vi "Galobal variable_TI.vi"() -> ()   [LabVIEW 2015]
panel:
  in  "Operator ID":string
  in  "Server":bool
  in  "Shift":T1
  out "Rework bit":bool
  out "Tracibility":bool
  in  "NG Count":u8
  in  "Shift  Change":string
  in  "User ID":string
  in  "Tier Value":dbl format="%0.03f"
  in  "Pokayoka Status":bool
  in  "LVDT Result":string
  in  "LVDTData(mm)":string
  in  "Load  Actual(N)":string
  in  "Rpt Delete":bool
  in  "Rpt Write":bool
  in  "Rpt Read":bool
  out "RSTC":string
  out "RSBC":string
  out "LBT":string
  out "Write data for model":string
  in  "Model trigger bit":bool
  out "RBT":string
  out "ng":bool
  out "ok":bool
  out "Reset":bool
  out "Emergency":bool
  out "Error":string[](array[string])
  in  "LOad Lvdt data":T2
  in  "Load Offset":dbl format="%0.03f"
  in  "DifssuerBARCPDE":string
  in  "LOAD NG":bool
  in  "BARCPDE":string
  in  "Camera Result":string
  in  "CAM Trigger":bool
  in  "LVDT Status":string
  in  "Load Status":string
  in  "Job ID":string
  in  "Load value":dbl format="%0.03f"
  in  "Load tear bit":bool
  in  "Running Model":string
  out "Sensor Data":T3 {"IL Sensor1_AI05" format="%0.02f"; "IL Sensor1_AI04" format="%0.02f"}
  in  "ILSensor Setting":T4
  in  "NI Comm.Error":bool
  in  "LVDT":dbl format="%0.03f"
  in  "Load Cell":dbl format="%0.03f"
  in  "Digital Output":bool[](array[boolean])
  in  "Auto Exit":bool
  in  "Slid Servo Home bit":bool
  in  "Call Home M2":bool
  in  "Call Home M1":bool
  in  "Barcode Lenght":i32
  in  "Barcode Scan Bit":bool
  in  "Barcode Data":string
  in  "Control Enable":bool
  in  "Stop M1":bool
  in  "Stop M2":bool
  in  "Programlist":string[](array[string])
  in  "STM Done Bit":bool
  in  "Offset_2":dbl
  in  "Offset_1":dbl
  in  "Slop _2":dbl
  in  "Slop_1":dbl
  out "Analoge Input":dbl[](array[numeric])
  out "AI_as DI":bool[](array[boolean])
  out "Manual DO":bool[](array[boolean])
  in  "Manual CMD":bool
  out "File Path":path[](array[path])
  out "Digital input":bool[](array[boolean])
  in  "User Name":string
  in  "Exit":bool
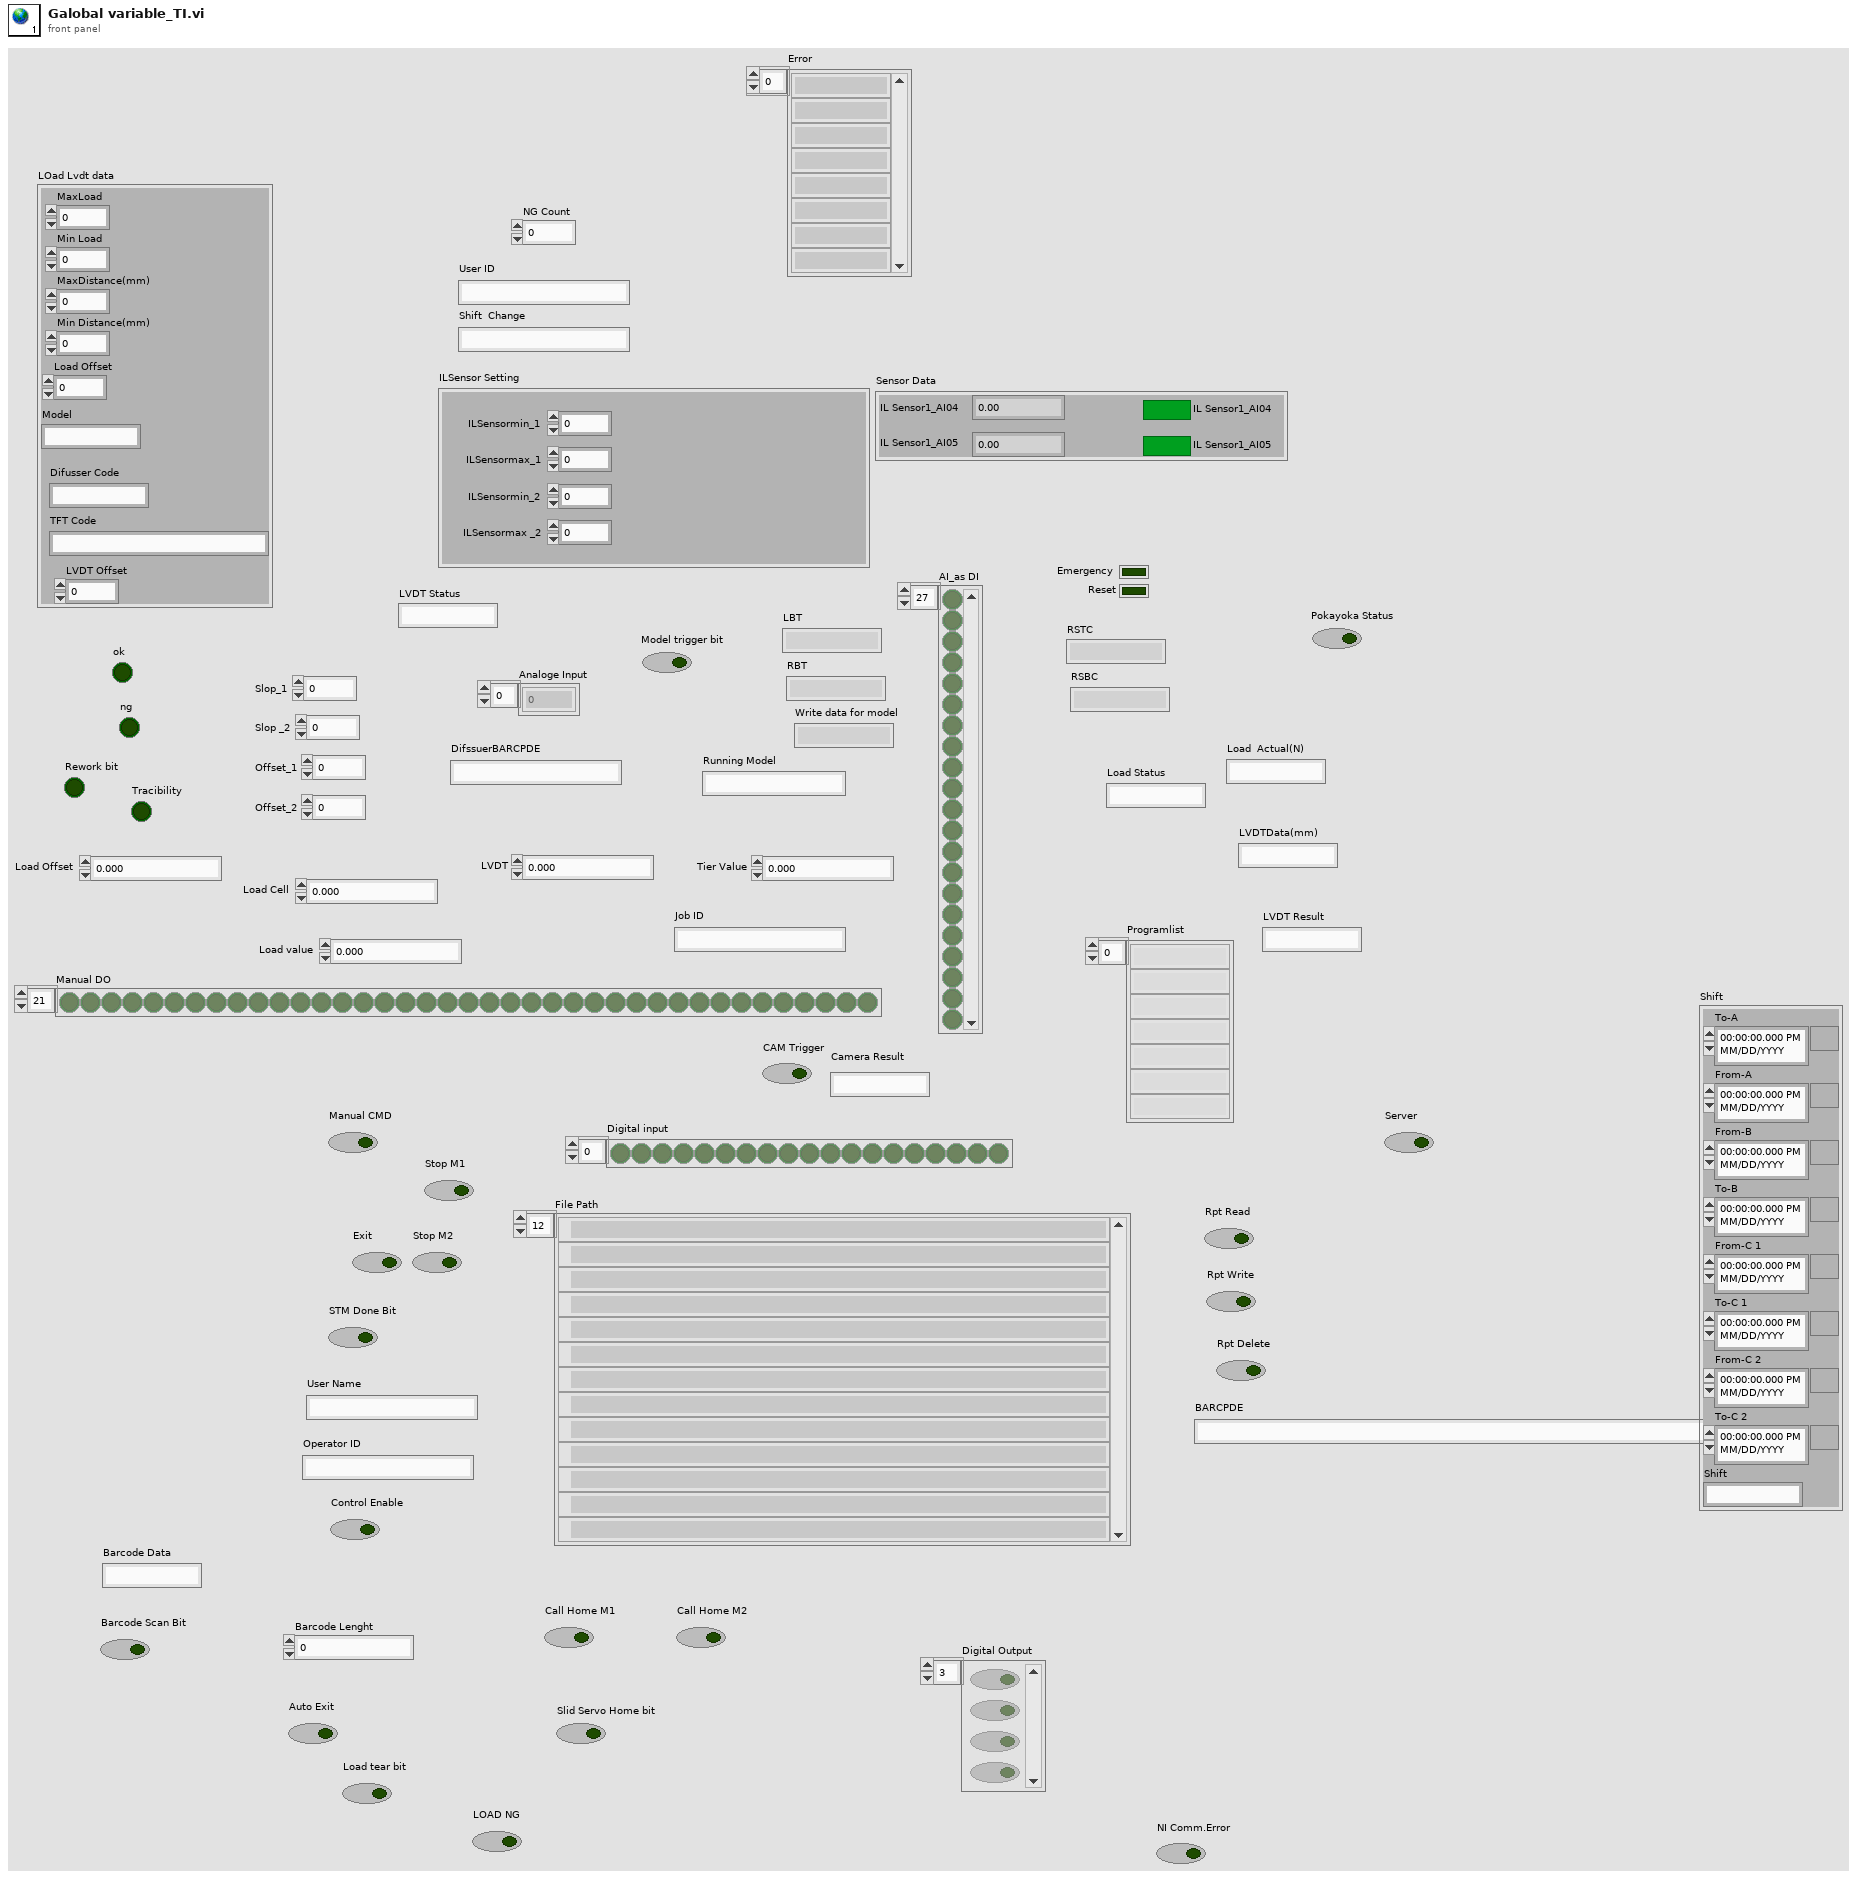
[diagram p1: front panel]
types:
  T1 = cluster{"To-A":timestamp, "From-A":timestamp, "From-B":timestamp, "To-B":timestamp, "From-C 1":timestamp, "To-C 1":timestamp, "From-C 2":timestamp, "To-C 2":timestamp, "Shift":string}
  T2 = cluster{"MaxLoad ":dbl, "Min Load":dbl, "MaxDistance(mm)":dbl, "Min Distance(mm)":dbl, "Load Offset":dbl, "Model":string, "Difusser Code":string, "TFT Code ":string, "LVDT Offset":dbl}
  T3 = cluster{"IL Sensor1_AI04":dbl, "IL Sensor1_AI05":dbl, "IL Sensor1_AI04":bool, "IL Sensor1_AI05":bool}
  T4 = cluster{"ILSensormax_1":dbl, "ILSensormin_1":dbl, "ILSensormax _2":dbl, "ILSensormin_2":dbl}
diagram:
